vi "LVFunction_Imop_SlopesPostProcessor_Apply Modulator.vi"(0 "HasoSlopes in":refnum<class "HasoSlopes.lvclass">, 5 "HasoSlopes OUT":refnum<class "HasoSlopes.lvclass">, 7 "filter":T1, 11 "error in (no error)":errorcluster) -> (4 "HasoSlopes out":refnum<class "HasoSlopes.lvclass">, 6 "HasoSlopes OUT 2":refnum<class "HasoSlopes.lvclass">, 15 "error out":errorcluster)   [LabVIEW 2020]
doc: "Modulates (multiply by a real factor between 0 and 1) some HasoSlopes\naberrations.\n\n<B>Slopes_inIn</B> : HasoSlopes object, modified by the processor if Slopes_out = NULL.\n<B>Slopes_inOut</B> : HasoSlopes object, modified by the processor if Slopes_out = NULL.\n<B>tiltx_modulation</B> : Value of x tilt modulation between 0 and 1.\n<B>tilty_modulation</B> : Value of y tilt modulation between 0 and 1.\n<B>curv_modulation</B> : Value of curvature modulation between 0 and 1.\n<B>astig0_modulation</B> : Value of 0 degree astigmatism modulation between 0 and 1.\n<B>astig45_modulation</B> : Value of 45 degree astigmatism modulation between 0 and 1.\n<B>others_modulation</B> : Value of all other aberrations modulation between 0 and 1.\n<B>Slopes_out</B> : processed HasoSlopes object if not NULL."
uses:
  HasoSlopes.lvclass
  SlopesPostProcessorList - Modulator.ctl
  LVClass_HasoSlopes Read HasoSlopes _ property.vi
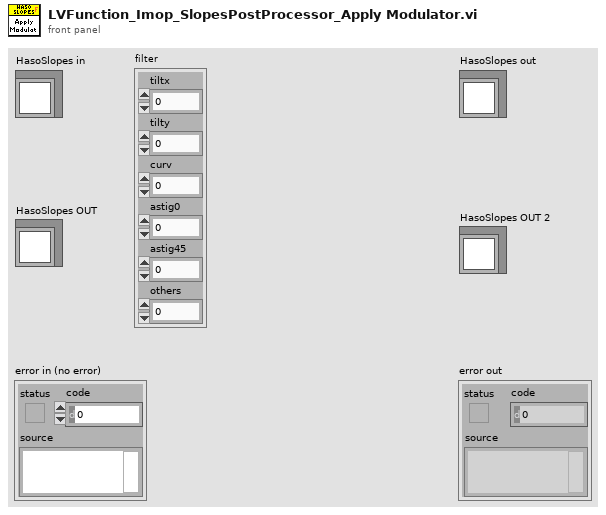
[diagram p1: front panel]
types:
  T1 = typedef "SlopesPostProcessorList - Modulator.ctl" = cluster{"tiltx":sgl, "tilty":sgl, "curv":sgl, "astig0":sgl, "astig45":sgl, "others":sgl}
  T2 = typedef "ClassID.ctl" = i64
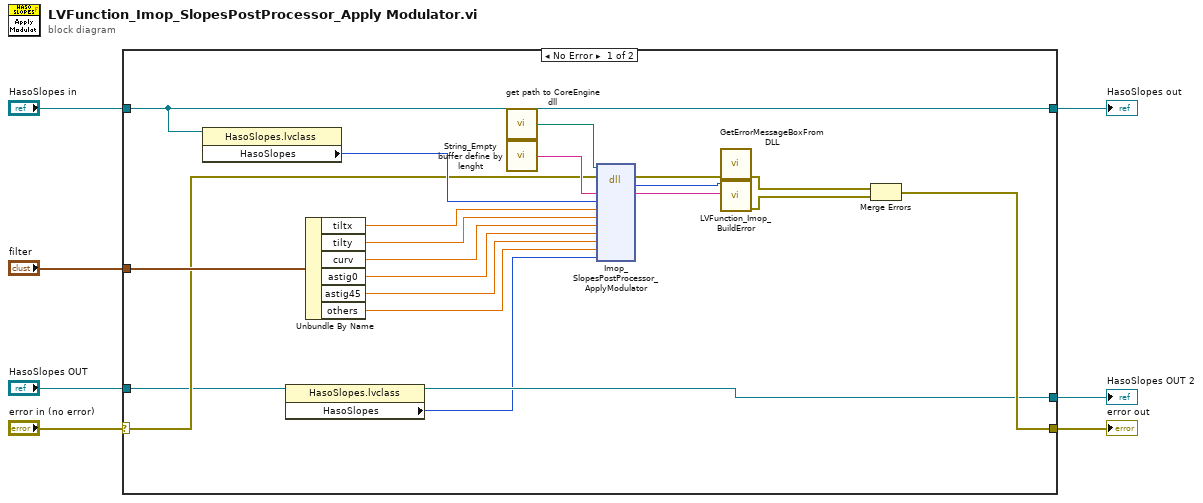
[diagram p0: block diagram]
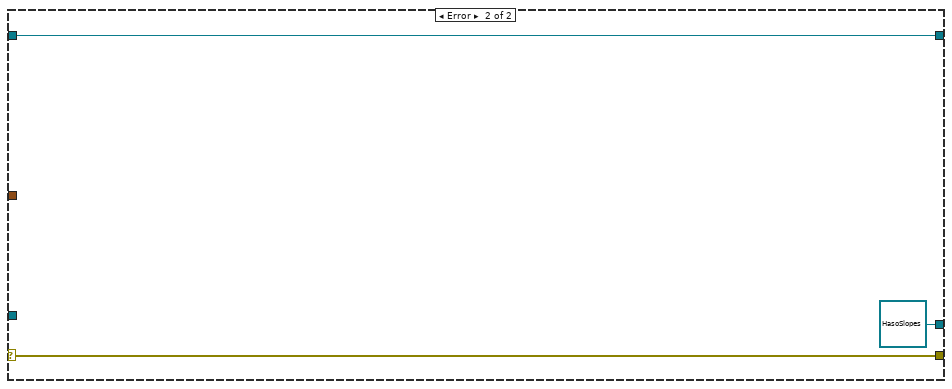
[diagram p2: hidden frame]
diagram:
  n1 = case shown="No Error" "error in (no error)" {
    selector: "error in (no error)" -> [w19 w31]
    tunnel: [w18 w31] -> w3
    tunnel: [w15 w30] -> w4
    tunnel: "HasoSlopes in" -> [w15 w30]
    tunnel: "filter" -> [w20 _]
    tunnel: "HasoSlopes OUT" -> [w17 _]
    tunnel: [w16 refnum<class "HasoSlopes.lvclass"> refnum ("HasoSlopes OUT")] -> w5
    frame No Error {
      n2 = property class="HasoSlopes.lvclass"(reference=w15) -> ("HasoSlopes"=w21:T2)  [unwired: 1 in, 2 out]
      n3 = property class="HasoSlopes.lvclass"(reference=w17) -> (reference out=w16:refnum<class "HasoSlopes.lvclass">, "HasoSlopes"=w8:T2)  [unwired: 1 in, 1 out]
      n4 = Unbundle By Name(w20) -> ("tiltx"=w14:sgl, "tilty"=w13:sgl, "curv"=w12:sgl, "astig0"=w11:sgl, "astig45"=w10:sgl, "others"=w9:sgl)
      n5 = call "get path to CoreEngine dll.vi"() -> ("path to wavekit library"=w22:path)  [unwired: 14 in, 1 out]
      n6 = call "String_Empty buffer define by lenght.vi"() -> ("Empty buffer"=w23:string)  [unwired: 1 in]
      n7 = dll-call lib="D:/FLE/0.Code/CoreEngine4_Suite/LV2011_interface/DLLs/c_interface_vc100.dll" fn="Imop_SlopesPostProcessor_ApplyModulator"(path in=w22, error in=w19, "Message"=w23, "SlopesPostProcessor"=w21, "tiltx"=w14, "tilty"=w13, "curv"=w12, "astig0"=w11, "astig45"=w10, "others"=w9, "HasoSlopes OUT"=w8) -> (error out=w24:errorcluster, "return type"=w25:i32, "Message"=w26:string)  [unwired: 9 in, 1 out]
      n8 = call "GetErrorMessageBoxFromDLL.vi"("error IN"=w24) -> ("error OUT"=w27:errorcluster)  [unwired: 10 in]
      n9 = call "LVFunction_Imop_BuildError.vi"("code"=w25, "String to Prepend to source (\"\")"=w26) -> ("error out"=w28:errorcluster)  [unwired: 13 in]
      n10 = Merge Errors(w27, w28) -> (w18:errorcluster)
    }
    frame Error {
    }
  }
  "error out" <- w3
  "HasoSlopes out" <- w4
  "HasoSlopes OUT 2" <- w5
